vi "Multi Goal Get.vi"() -> (0 "R Robot-Rel X":dbl, 1 "R Found?":bool, 2 "L Robot-Rel X":dbl, 3 "L Found?":bool, 4 "R Dist":dbl, 5 "L Dist":dbl, 6 "R Target":T1, 7 "L Target":T1)   [LabVIEW 2013]
uses:
  Common Code/Goal Info.ctl
  Common Code/Vision Packet.ctl
  <vilib>/Rock Robotics/WPI/DriverStation/WPI_DriverStationRobotMode2.ctl
  Robot Global Data.vi
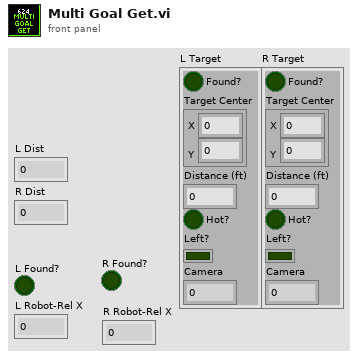
[diagram p1: front panel]
types:
  T1 = typedef "Goal Info.ctl" = cluster{"Found?":bool, "Target Center":cluster{"X":dbl, "Y":dbl}, "Distance (ft)":dbl, "Hot?":bool, "Left?":bool, "Camera":i16}
  T2 = typedef "Vision Packet.ctl" = cluster{"Gyro":dbl, "Vision Target":T1, "Timestamp":u32, "Left Goal":T1, "Right Goal":T1}
  T3 = typedef "WPI_DriverStationRobotMode2.ctl" = enum16{"Autonomous Disabled", "Autonomous Enabled", "Teleop Disabled", "Teleop Enabled", "Timeout", "Finish", "Test Disabled", "Test Enabled"}
  T4 = typedef "Dashboard UDP Packet.ctl" = cluster{"Camera":T5, "Gyro":T6, "Encoder":T8, "Auto Shift":T9, "Auton":T10, "Drive/Ramp X":dbl, "Drive/Ramp Y":dbl, "Drive/Battery Cutoff":dbl, "Pressure/Compressor Min Voltage":dbl, "Pressure/Compressor Delay":dbl, "Controller/Strafe Correction":bool, "Shooter":T11, "Rollers":T12, "Abort":bool, "Finish":bool, "IR Halo Sustain Time":dbl, "Disable Compressor":bool}
  T5 = typedef "Camera Controls.ctl" = cluster{"Camera/View Angle X":dbl, "Camera/Goal Track Timeout":dbl, "Camera/View Angle Y":dbl, "Camera/Goal Exposure":dbl, "Camera/Vision Receive Timeout":dbl, "Camera/Offset 1":dbl, "Camera/Offset 2":dbl}
  T6 = typedef "Gyro Controls.ctl" = cluster{"Gyro/Angle Tolerance":dbl, "Gyro/Steer Closeness Threshold":dbl, "Steer PID":T7, "Steer Close PID":T7}
  T7 = typedef "PID Params.ctl" = cluster{"max":dbl, "min":dbl, "P":dbl, "I":dbl, "D":dbl}
  T8 = typedef "Encoder Controls.ctl" = cluster{"Encoders/Reset":bool, "Encoders/Omni Constant":dbl, "Encoders/Omni Tick Constant":dbl, "Encoders/Left Constant":dbl, "Encoders/Right Constant":dbl, "Encoders/Right Tick Constant":dbl}
  T9 = typedef "Auto Shift Controls.ctl" = cluster{"AutoShift/Upshift Throttle Accel":dbl, "AutoShift/Speed Threshold":dbl, "AutoShift/Upshift Throttle":dbl, "AutoShift/Upshift Accel":dbl, "AutoShift/Downshift Accel":dbl, "AutoShift/Downshift Throttle":dbl, "AutoShift/Delay":dbl, "AutoShift/Enabled":bool}
  T10 = typedef "Auton Controls.ctl" = cluster{"Auton/Left Shoot X-Coord":dbl, "Auton/Right Shoot X-Coord":dbl, "DistDrive/Distance Stop Threshold":dbl, "DistDrive/Max Stop Speed":dbl, "Auton/Back Piston Time":dbl, "Auton/Manual Hot":bool, "Auton/Manual Hot Right":bool, "Default X PID":T7, "Default Y PID":T7}
  T11 = typedef "Shooter Controls.ctl" = cluster{"Shooter/Reset Time":dbl, "Shooter/Release Delay":dbl, "Shooter/Pressure Steady Time":dbl, "Shooter/Misfire Delay":dbl, "Shooter/Ball Settle Time":dbl, "Shooter/Line IR Delay":dbl, "Pressure/Upper PSI Time":dbl, "Pressure/Lower PSI Time":dbl, "Shooter/Punch Delay":dbl, "Shooter/Target Pressure":dbl, "Pressure/Line B":dbl, "Pressure/Line M":dbl, "Pressure/Shooter M":dbl, "Pressure/Shooter B":dbl, "Halo Time":dbl, "Soft Release Delay":dbl, "Soft Unpin Delay":dbl, "Soft Shoot Delay":dbl}
  T12 = typedef "Roller Controls.ctl" = cluster{"Roller/Load IRs Verify Time":dbl, "Roller/Center IR Latch Time":dbl, "Roller/Speed Front":dbl, "Roller/Speed Back":dbl, "Roller/Entry Timeout":dbl, "Roller/To Center Timeout":dbl, "Roller/Sustain Time":dbl, "Roller/Verify Center Time":dbl}
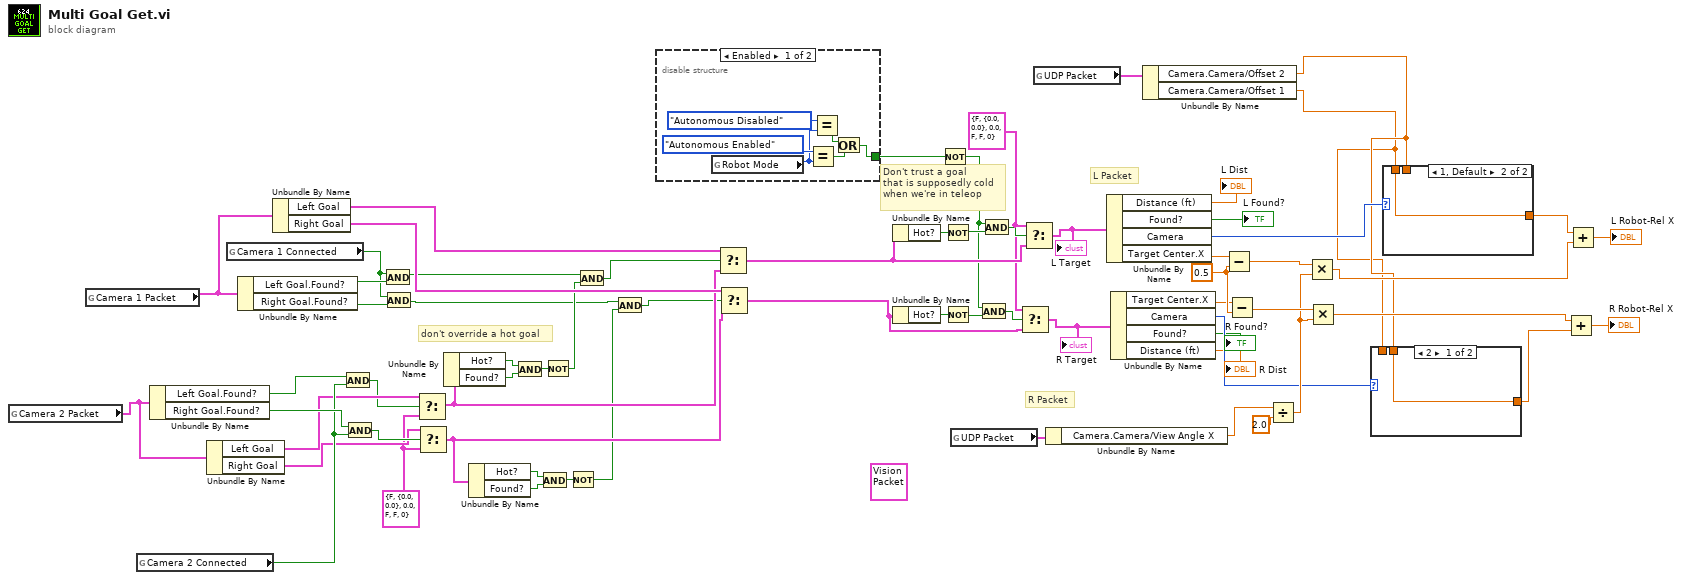
[diagram p0: block diagram]
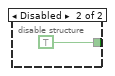
[diagram p2: hidden frame]
diagram:
  w24 = T1 {"Found?"=FALSE, "Target Center"={"X"=0.0, "Y"=0.0}, "Distance (ft)"=0.0, "Hot?"=FALSE, "Left?"=FALSE, "Camera"=0} ("input cluster")
  w50 = 0.5 ("y")
  w52 = T1 {"Found?"=FALSE, "Target Center"={"X"=0.0, "Y"=0.0}, "Distance (ft)"=0.0, "Hot?"=FALSE, "Left?"=FALSE, "Camera"=0} ("f")
  (unwired) T2 {"Gyro"=0.0, "Vision Target"={"Found?"=FALSE, "Target Center"={"X"=0.0, "Y"=0.0}, "Distance (ft)"=0.0, "Hot?"=FALSE, "Left?"=FALSE, "Camera"=0}, "Timestamp"=0, "Left Goal"={"Found?"=FALSE, "Target Center"={"X"=0.0, "Y"=0.0}, "Distance (ft)"=0.0, "Hot?"=FALSE, "Left?"=FALSE, "Camera"=0}, "Right Goal"={"Found?"=FALSE, "Target Center"={"X"=0.0, "Y"=0.0}, "Distance (ft)"=0.0, "Hot?"=FALSE, "Left?"=FALSE, "Camera"=0}} ("f")
  # "don't override a hot goal"
  # "Don't trust a goal\nthat is supposedly cold\nwhen we're in teleop"
  # "R Packet"
  # "L Packet"
  n1 = global read "Robot Global Data.vi" "Camera 2 Packet"() -> (w55:T2)
  n2 = global read "Robot Global Data.vi" "Camera 1 Packet"() -> (w58:T2)
  n3 = global read "Robot Global Data.vi" "Camera 2 Connected"() -> (w61:bool)
  n4 = Unbundle By Name(w55) -> ("Left Goal.Found?"=w63:bool, "Right Goal.Found?"=w62:bool)
  n5 = Unbundle By Name(w55) -> ("Left Goal"=w54:T1, "Right Goal"=w53:T1)
  n6 = global read "Robot Global Data.vi" "Camera 1 Connected"() -> (w65:bool)
  n7 = Unbundle By Name(w58) -> ("Left Goal.Found?"=w66:bool, "Right Goal.Found?"=w64:bool)
  n8 = Unbundle By Name(w58) -> ("Left Goal"=w57:T1, "Right Goal"=w56:T1)
  n9 = And(x=w63, y=w61) -> (x .and. y?=w20:bool)
  n10 = And(x=w62, y=w61) -> (x .and. y?=w60:bool)
  n11 = And(x=w65, y=w66) -> (x .and. y?=w14:bool)
  n12 = And(x=w65, y=w64) -> (x .and. y?=w8:bool)
  n13 = Select(t=w54, s=w20, f=w52) -> (s? t:f=w19:T1)
  n14 = Select(t=w53, s=w60, f=w52) -> (s? t:f=w9:T1)
  n15 = Unbundle By Name(w19) -> ("Hot?"=w18:bool, "Found?"=w17:bool)
  n16 = Unbundle By Name(w9) -> ("Hot?"=w10:bool, "Found?"=w11:bool)
  n17 = And(x=w18, y=w17) -> (x .and. y?=w16:bool)
  n18 = And(x=w10, y=w11) -> (x .and. y?=w12:bool)
  n19 = Not(x=w16) -> (.not. x?=w15:bool)
  n20 = Not(x=w12) -> (.not. x?=w7:bool)
  n21 = And(x=w14, y=w15) -> (x .and. y?=w13:bool)
  n22 = And(x=w8, y=w7) -> (x .and. y?=w6:bool)
  n23 = disable-structure shown="Enabled" {
    disable-tunnel: [w67 TRUE] -> w21
    frame Enabled {
      n24 = global read "Robot Global Data.vi" "Robot Mode"() -> (w71:T3)
      n25 = Equal?(x=WPI_DriverStationRobotMode2."Autonomous Enabled", y=w71) -> (x = y?=w69:bool)
      n26 = Equal?(x=WPI_DriverStationRobotMode2."Autonomous Disabled", y=w71) -> (x = y?=w68:bool)
      n27 = Or(x=w68, y=w69) -> (x .or. y?=w67:bool)
    }
    frame Disabled {
    }
  }
  n28 = Select(t=w57, s=w13, f=w19) -> (s? t:f=w30:T1)
  n29 = Select(t=w56, s=w6, f=w9) -> (s? t:f=w23:T1)
  n30 = Unbundle By Name(w30) -> ("Hot?"=w33:bool)
  n31 = Unbundle By Name(w23) -> ("Hot?"=w28:bool)
  n32 = Not(x=w21) -> (.not. x?=w25:bool)
  n33 = Not(x=w33) -> (.not. x?=w32:bool)
  n34 = Not(x=w28) -> (.not. x?=w27:bool)
  n35 = global read "Robot Global Data.vi" "UDP Packet"() -> (w2:T4)
  n36 = And(x=w25, y=w27) -> (x .and. y?=w26:bool)
  n37 = And(x=w25, y=w32) -> (x .and. y?=w31:bool)
  n38 = Select(t=w24, s=w26, f=w23) -> (s? t:f=w22:T1)
  "R Target" <- w22
  n39 = Select(t=w24, s=w31, f=w30) -> (s? t:f=w29:T1)
  "L Target" <- w29
  n40 = global read "Robot Global Data.vi" "UDP Packet"() -> (w5:T4)
  n41 = Unbundle By Name(w2) -> ("Camera.Camera/View Angle X"=w1:dbl)
  n42 = Unbundle By Name(w29) -> ("Distance (ft)"=→"L Dist":dbl, "Found?"=→"L Found?":bool, "Camera"=w45:i16, "Target Center.X"=w51:dbl)
  n43 = Unbundle By Name(w22) -> ("Target Center.X"=w49:dbl, "Camera"=w44:i16, "Found?"=→"R Found?":bool, "Distance (ft)"=→"R Dist":dbl)
  n44 = Unbundle By Name(w5) -> ("Camera.Camera/Offset 2"=w4:dbl, "Camera.Camera/Offset 1"=w3:dbl)
  n45 = Subtract(x=w51, y=w50) -> (x-y=w48:dbl)
  n46 = Subtract(x=w49, y=w50) -> (x-y=w47:dbl)
  n47 = Divide(x=w1, y=2.0) -> (x/y=w46:dbl)
  n48 = Multiply(x=w48, y=w46) -> (x*y=w42:dbl)
  n49 = Multiply(x=w47, y=w46) -> (x*y=w41:dbl)
  n50 = case shown="2" w44 {
    tunnel: w3 -> [_ w75]
    tunnel: w4 -> [w74 _]
    tunnel: [w74 w75] -> w40
    frame 2 {
    }
    frame 1, Default {
    }
  }
  n51 = case shown="1, Default" w45 {
    tunnel: w3 -> [_ w77]
    tunnel: w4 -> [w76 _]
    tunnel: [w76 w77] -> w43
    frame 2 {
    }
    frame 1, Default {
    }
  }
  n52 = Add(x=w41, y=w40) -> (x+y=→"R Robot-Rel X":dbl)
  n53 = Add(x=w43, y=w42) -> (x+y=→"L Robot-Rel X":dbl)
